vi "SwitchSystem.vi"   [LabVIEW 2019]
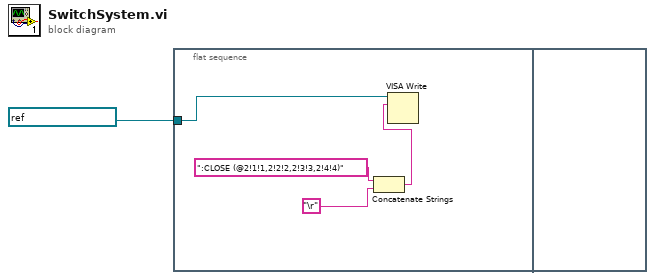
[diagram p0: block diagram]
diagram:
  n1 = flat-sequence {
    tunnel: refnum<visa-resource-name> "GPIB0::7::INSTR" ("VISA resource name") -> [w5]
    frame #0 {
      n2 = Concatenate Strings(":CLOSE (@2!1!1,2!2!2,2!3!3,2!4!4)", "\r") -> (w3:string)
      n3 = VISA Write(VISA resource name=w5, write buffer=w3) -> ()  [unwired: 1 in, 3 out]
    }
    frame #1 {
    }
  }
